vi "Siglent SDG X Series Standard Waveform-mod.vi"() -> ()   [LabVIEW 2020]
doc: "This example shows how to generate a standard waveform."
uses:
  <instrlib>/Siglent SDG X Series/Siglent SDG X Series.lvlib
panel:
  in  "Duty Cycle (50.0%)":dbl=99.0 min=20.0 max=99.0 format="%.1g"
  in  "Amplitude (1.0 Vpp)":dbl=5.0 format="%#.3f"
  in  "VISA resource name":refnum<visa-resource-name>
  in  "DC Offset (0.00 V)":dbl=-2.5
  in  "Frequency (1000 Hz)":dbl=100.0 format="%#.6g"
  in  "Channel (1:Channel 1)":i32(ring)=1 items=["Channel 1"=1, "Channel 2"=2]
  in  "Waveform Function (0: Sine)":u16(ring)=1 items=["Sine", "Square", "Triangle", "DC", "Pulse", "Arb"]
  # "WARNING. RUN ONLY WHEN LASER IS SHUTTERED"
  # "(c) 2017 SIGLENT TECHNOLOGIES CO.,LTD. ALL RIGHTS RESERVED."
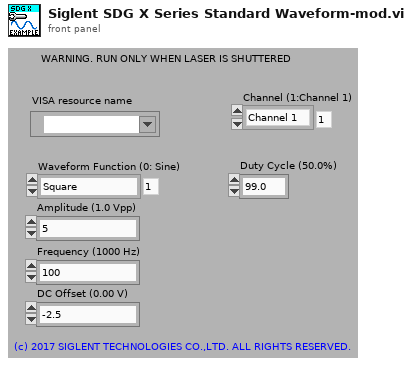
[diagram p1: front panel]
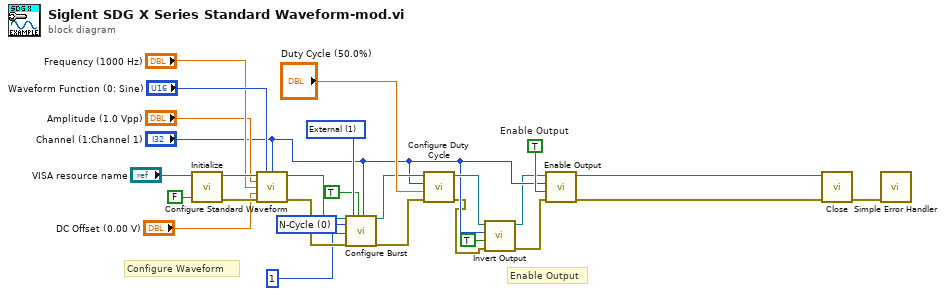
[diagram p0: block diagram]
diagram:
  w8 = u16 0 items=["N-Cycle", "Infinite"] ("Burst Cycle (0: N-Cycle)")
  w10 = u16 1 items=["Internal", "External", "Manual"] ("Trigger Source (0: Internal)")
  w22 = TRUE  # Enable Output
  # "Enable Output"
  # "Configure Waveform"
  n1 = call <instrlib>:"Initialize.vi"("Reset (True)"=FALSE, "VISA resource name"="VISA resource name") -> ("error out"=w26:errorcluster, "VISA resource name out"=w27:refnum<visa-resource-name>)  [unwired: 8 in]
  n2 = call <instrlib>:"Configure Standard Waveform.vi"("VISA resource name"=w27, "Waveform Function (0: Sine)"="Waveform Function (0: Sine)", "Channel (1:Channel 1)"="Channel (1:Channel 1)", "Amplitude (1.0 Vpp)"="Amplitude (1.0 Vpp)", "Frequency (1000 Hz)"="Frequency (1000 Hz)", "DC Offset (0.00 V)"="DC Offset (0.00 V)", "error in (no error)"=w26) -> ("VISA resource name out"=w14:refnum<visa-resource-name>, "error out"=w13:errorcluster)  [unwired: 7 in]
  n3 = call <instrlib>:"Configure Burst.vi"("VISA resource name"=w14, "Burst Cycle (0: N-Cycle)"=w8, "Number of Cycles (1)"=1, "error in (no error)"=w13, "Trigger Source (0: Internal)"=w10, "Enable Burst Mode (T:Enable)"=TRUE, "Channel (1:Channel 1)"="Channel (1:Channel 1)") -> ("VISA resource name out"=w11:refnum<visa-resource-name>, "error out"=w12:errorcluster)  [unwired: 11 in]
  n4 = call <instrlib>:"Configure Duty Cycle.vi"("error in (no error)"=w12, "Duty Cycle (50.0%)"="Duty Cycle (50.0%)", "Channel (1:Channel 1)"="Channel (1:Channel 1)", "VISA resource name"=w11) -> ("error out"=w2:errorcluster, "VISA resource name out"=w6:refnum<visa-resource-name>)  [unwired: 6 in]
  n5 = call <instrlib>:"Invert Output.vi"("error in (no error)"=w2, "Enable Channel Invert (F: Disable)"=TRUE, "Channel (1:Channel 1)"="Channel (1:Channel 1)", "VISA resource name"=w6) -> ("error out"=w1:errorcluster, "VISA resource name out"=w4:refnum<visa-resource-name>)  [unwired: 6 in]
  n6 = call <instrlib>:"Enable Output.vi"("error in (no error)"=w1, "Enable Output (T: Enable)"=w22, "Channel (1:Channel 1)"="Channel (1:Channel 1)", "VISA resource name"=w4) -> ("error out"=w23:errorcluster, "VISA resource name out"=w24:refnum<visa-resource-name>)  [unwired: 6 in]
  n7 = call <instrlib>:"Close.vi"("error in (no error)"=w23, "VISA resource name"=w24) -> ("error out"=w25:errorcluster)  [unwired: 9 in]
  n8 = call <vilib>:"Simple Error Handler.vi"("error in (no error)"=w25) -> ()  [unwired: 4 in, 5 out]
